vi "Read FftView.vi"(8 "error in (no error)":errorcluster, 11 "FFT in":refnum<class "FFT.lvclass">) -> (0 "error out":errorcluster, 2 "FftView":T1, 3 "FFT out":refnum<class "FFT.lvclass">)   [LabVIEW 2014, in "AnalysisPlugins.lvlib" / "FFT.lvclass"]
uses:
  FFT.lvclass
  Typedefs/FftView.ctl
  FFT.lvclass/FFT.ctl
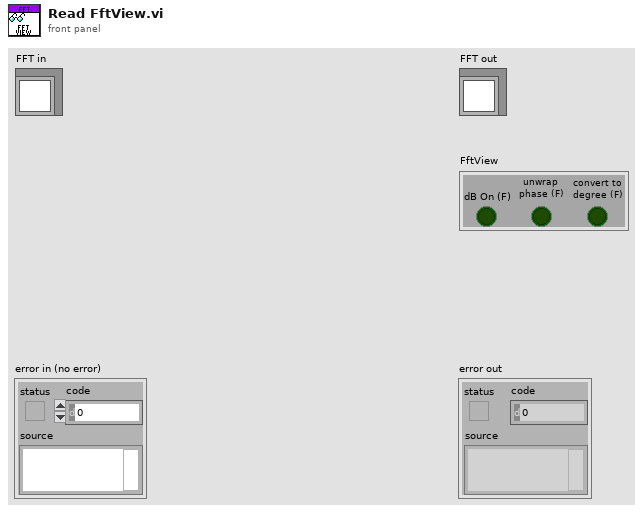
[diagram p1: front panel]
types:
  T1 = typedef "AnalysisPlugins.lvlib/FFT.lvclass/FftView.ctl" = cluster{"dB On (F)":bool, "unwrap phase (F)":bool, "convert to degree (F)":bool}
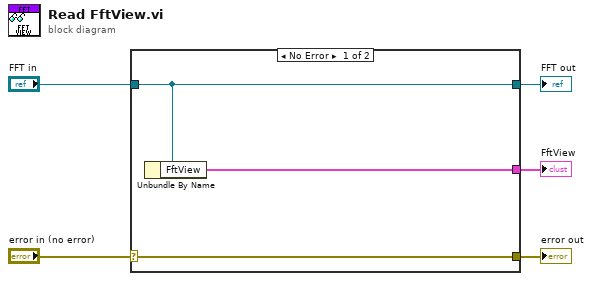
[diagram p0: block diagram]
diagram:
  n1 = case shown="No Error" "error in (no error)" {
    selector: "error in (no error)" -> [w8 w9]
    tunnel: [w8 w9] -> w4
    tunnel: [w7 w10] -> w2
    tunnel: "FFT in" -> [w7 w10]
    tunnel: [w6 _] -> w1
    frame No Error {
      n2 = Unbundle By Name(w7) -> ("FftView"=w6:T1)
    }
    frame Error {
    }
  }
  "error out" <- w4
  "FFT out" <- w2
  "FftView" <- w1
